vi "BuildScansMeasArrays.vi"(0 "Scans in":T3(array[cluster]) {"Stop" format="%.9f"; "Start" format="%.9f"}) -> (1 "Scans out":T3(array[cluster]) {"Stop" format="%.9f"; "Start" format="%.9f"}, 2 "ScanStep":i32[](array[numeric]), 3 "ScanSizes":i32[](array[numeric]))   [LabVIEW 2017]
uses:
  ScanTarget.ctl
  ScanPara.ctl
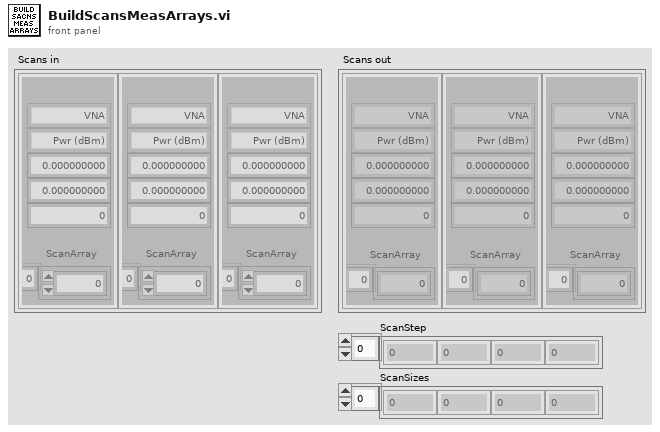
[diagram p1: front panel]
types:
  T1 = typedef "ScanTarget.ctl" = enum16{"VNA", "Refrigerator"}
  T2 = typedef "ScanPara.ctl" = enum16{"Freq (GHz)", "Pwr (dBm)", "Temp (K)", "N.A."}
  T3 = cluster{"Target":T1, "Parameter":T2, "Start":dbl, "Stop":dbl, "#Steps":u32, "ScanArray":dbl[]}[]
  T4 = cluster{"Target":T1, "Parameter":T2, "Start":dbl, "Stop":dbl, "#Steps":u32, "ScanArray":dbl[]}
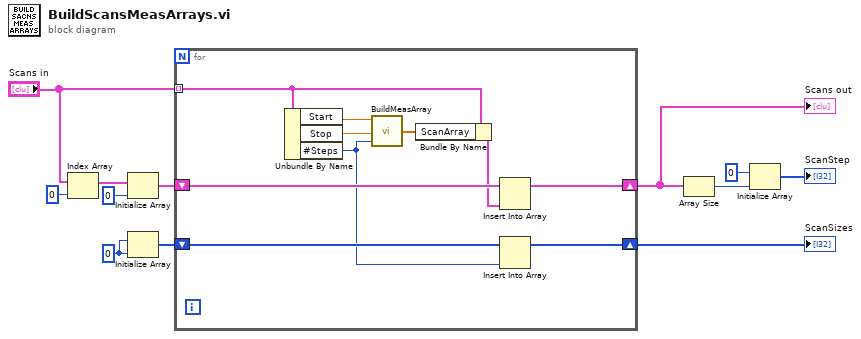
[diagram p0: block diagram]
diagram:
  w4 = 0 ("dimension size")
  n1 = Index Array(array="Scans in", index=0) -> (element=w10:T4)
  n2 = Initialize Array(w10, 0 ("dimension size")) -> (w9:T3)
  n3 = Initialize Array(w4, w4) -> (w12:i32[])
  n4 = for {
    shift-right: [w22] -> w1
    shift-left: w9 -> [w19]
    shift-right: [w20] -> w11
    shift-left: w12 -> [w21]
    tunnel: "Scans in" -> [w18] mode=indexing
    n5 = Unbundle By Name(w18) -> ("Start"=w15:dbl, "Stop"=w13:dbl, "#Steps"=w14:u32)
    n6 = call "BuildMeasArray.vi"("#Steps"=w14, "Stop"=w13, "Start"=w15) -> ("MeasArray"=w17:dbl[])
    n7 = Bundle By Name(cluster=w18, "ScanArray"=w17) -> (w16:T4)
    n8 = Insert Into Array(array=w19, new element=w16) -> (w22:T3)  [unwired: 1 in]
    n9 = Insert Into Array(array=w21, new element=w14) -> (w20:i32[])  [unwired: 1 in]
  }
  "ScanSizes" <- w11
  "Scans out" <- w1
  n10 = Array Size(array=w1) -> (size(s)=w8:i32)
  n11 = Initialize Array(0, w8) -> (→"ScanStep":i32[])
